vi "Write N.vi"(8 "error in (no error)":errorcluster, 10 "N":dbl, 11 "Online_SNR in":refnum<class "Online_SNR.lvclass">) -> (0 "error out":errorcluster, 3 "Online_SNR out":refnum<class "Online_SNR.lvclass">)   [LabVIEW 2021, in "Online_SNR.lvclass"]
uses:
  Online_SNR.lvclass
  Online_SNR.lvclass/Online_SNR.ctl
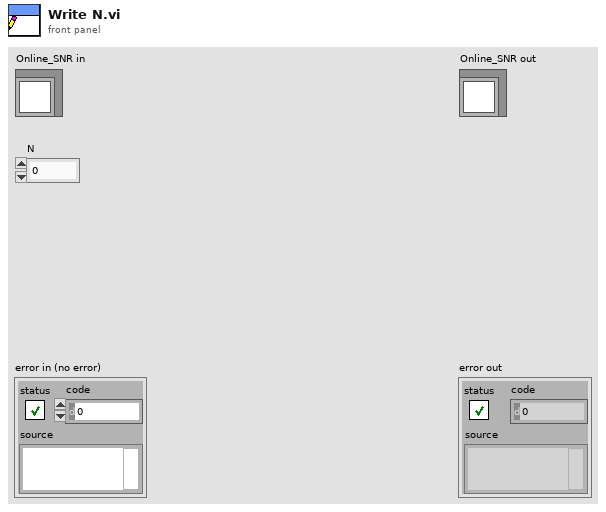
[diagram p1: front panel]
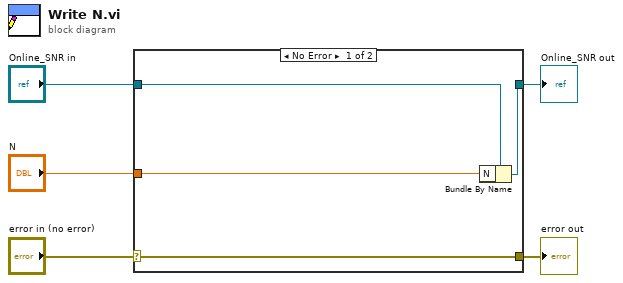
[diagram p0: block diagram]
diagram:
  n1 = case shown="No Error" "error in (no error)" {
    selector: "error in (no error)" -> [w9 w10]
    tunnel: [w9 w10] -> w4
    tunnel: [w7 w11] -> w2
    tunnel: "Online_SNR in" -> [w8 w11]
    tunnel: "N" -> [w6 _]
    frame No Error {
      n2 = Bundle By Name(cluster=w8, "N"=w6) -> (w7:refnum<class "Online_SNR.lvclass">)
    }
    frame Error {
    }
  }
  "error out" <- w4
  "Online_SNR out" <- w2
